vi "stim.vi"() -> ()   [LabVIEW 2010]
uses:
  <vilib>/DAQmx/write.llb/DAQmx Write (Digital Bool 1Line 1Point).vi
  Fear Conditioning/GlobalFear.vi
  <vilib>/imath/engines/lvmath2/RunTimeEngine/ErrorHandling/NIMS_Finalize Error.vi
  <vilib>/imath/engines/lvmath2/RunTimeEngine/NodeEndStatement/NIMS_NodeEndStatement_Get Vector.vi
  <instcachedir>/0/NIMS_NodeEndStatement_Get Vector_F420F1081A35401FA339BC91980782B0.lvgen/NIMS_NodeEndStatement_Get Vector_F420F1081A35401FA339BC91980782B0_002.vi
  <vilib>/imath/engines/lvmath/Functions/Error Handling/MergeErrorsWrapper.vi
  <vilib>/imath/engines/lvmath2/RunTimeEngine/NodeEndStatement/NIMS_NodeEndStatement_Output.vi
  <instcachedir>/0/NIMS_NodeEndStatement_Output_53EC0D466D134D7ABD903AC30B43404B.lvgen/NIMS_NodeEndStatement_Output_53EC0D466D134D7ABD903AC30B43404B_004.vi
  <instcachedir>/0/NIMS_NodeEndStatement_Output_53EC0D466D134D7ABD903AC30B43404B.lvgen/NIMS_NodeEndStatement_Output_53EC0D466D134D7ABD903AC30B43404B_005.vi
  <vilib>/imath/engines/lvmath2/RunTimeEngine/RangeToken/NIMS_Range.vi
  <instcachedir>/0/NIMS_Range_1C63927E4E474DADACDA97C3F2261A11.lvgen/NIMS_Range_1C63927E4E474DADACDA97C3F2261A11_000.vi
  <vilib>/imathl/engines/lvmath/Functions/Error Handling/Create Error.vi
  <vilib>/imath/engines/lvmath2/RunTimeEngine/BuiltInFunctions/repeatmx/NIMS_repeatmx(GM, I32, I32).vi
  <instcachedir>/0/NIMS_repeatmx(GM, I32, I32)_69DEE8FEFC4F4D9AB51BA55E85245ECE.lvgen/NIMS_repeatmx(GM, I32, I32)_69DEE8FEFC4F4D9AB51BA55E85245ECE_004.vi
  <vilib>/imath/engines/lvmath2/RunTimeEngine/BuiltInFunctions/randpermutation/NIMS_randpermutation.vi
  <vilib>/imath/engines/lvmath2/RunTimeEngine/VariableToken/Read/NIMS_Get Elements - SorM(_) - Check.vi
  <instcachedir>/0/NIMS_Get Elements - SorM(_) - Check_404BE36992094B78AAADB7BD5278D7E3.lvgen/NIMS_Get Elements - SorM(_) - Check_404BE36992094B78AAADB7BD5278D7E3_006.vi
  <vilib>/daqmx/miscellaneous.llb/DAQmx Fill In Error Info.vi
  <vilib>/measure/NI_MABase.lvlib
panel:
  out "Audio":bool
  in  "Audio\nSafety":bool=TRUE caption="Audio"
  out "Shock":bool
  out "Counter":dbl
  out "Elapsed Time":dbl format="%#_3g"
  out "Copleted":bool
  out "Trigger":bool
  out "Current Stim":dbl
  out "Audio\nDuration":dbl
  out "ITI":dbl
  out "Pattern \nFrequency":dbl
  out "Frequency":dbl
  out "Audio\nDelay":dbl
  out "Shock \nDuration":dbl=-1.0
  out "Shock\nDelay":dbl=-1.0
  out "raw stim":dbl
  out "Now Showing":string
  out "Dimentions":dbl
  out "expInd":dbl[](array[numeric])
  out "Stim":dbl[](array[numeric])
  out "Sum":dbl
  in  "Shock \nSafety":bool caption="Audio"
  in  "Stimuli":string[](array[combo])
  in  "Start 2":bool caption="Start"
  in  "Array 3":dbl[][](array[numeric])
  in  "Cluster 3":T1
  out "Stimulus Parameters":string[](array[string])
  in  "stop 2":bool
  # "Audio Duration"
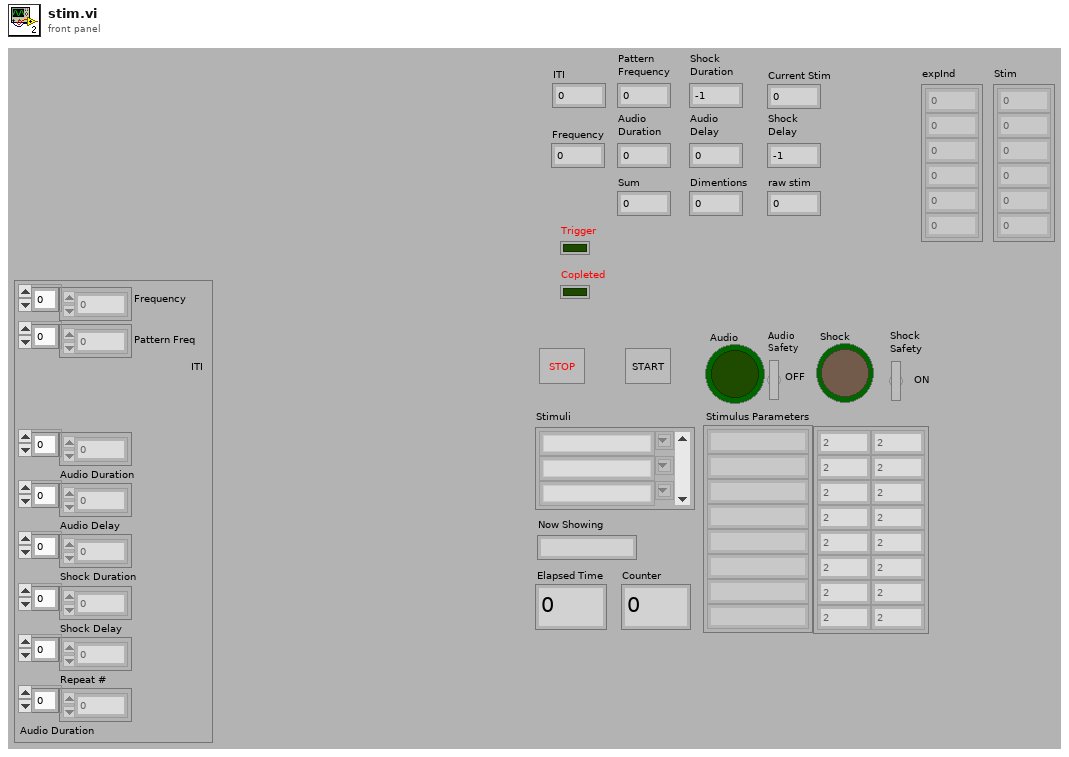
[diagram p1: front panel]
types:
  T1 = cluster{"Frequency":dbl[], "Pattern Freq":dbl[], "ITI":dbl[], "Audio Duration":dbl[], "Audio Delay":dbl[], "Shock Duration":dbl[], "Shock Delay":dbl[], "Repeat #":dbl[]}
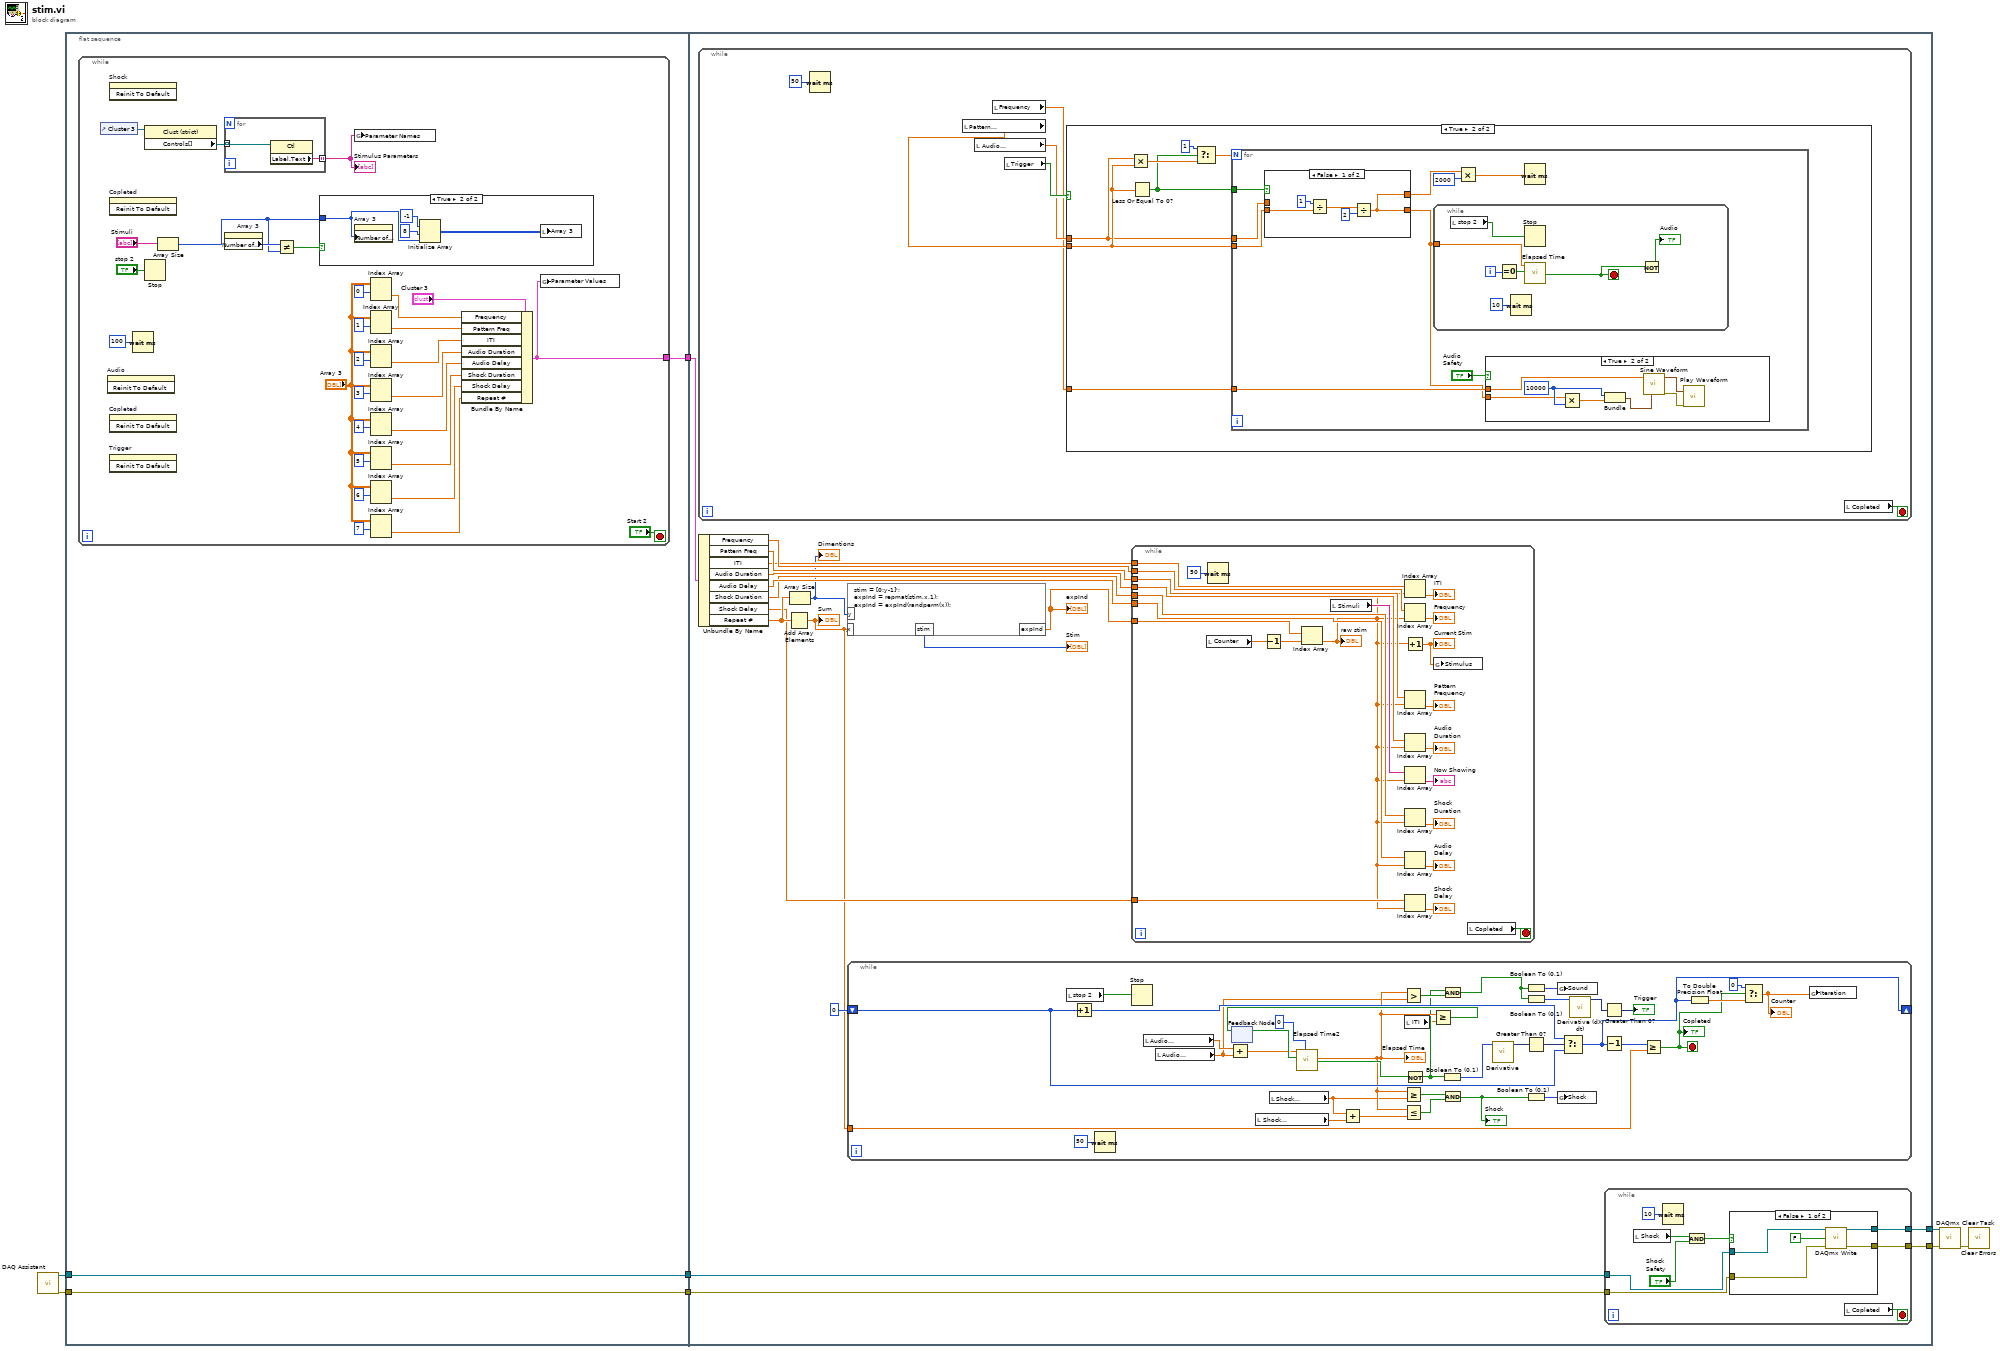
[diagram p0: block diagram]
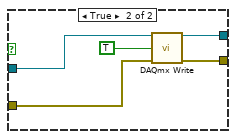
[diagram p3: hidden frame]
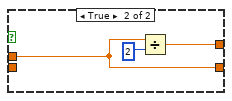
[diagram p6: hidden frame]
diagram:
  n1 = call "DAQ Assistant"() -> ("task out"=w4:refnum<k21>, "error out"=w3:errorcluster)  [unwired: 18 in]
  n2 = flat-sequence {
    tunnel: [w11] -> w8
    tunnel: w4 -> [w10]
    tunnel: [w10] -> w7
    tunnel: [w9] -> w6
    tunnel: w3 -> [w9]
    tunnel: w8 -> [w62]
    tunnel: [w50] -> w5
    tunnel: w7 -> [w49]
    tunnel: w6 -> [w48]
    tunnel: [w47] -> w2
    frame #0 {
      n3 = while {
        tunnel: [w14] -> w11
        stop <- "Start 2" stop-if-true
        n4 = control-ref of="Cluster 3"() -> (w17:refnum<vi>)
        n5 = invoke on="Audio" class="Bool (strict)" method="Reinit To Default"() -> ()  [unwired: 3 in, 3 out]
        n6 = invoke on="Shock" class="Bool (strict)" method="Reinit To Default"() -> ()  [unwired: 3 in, 3 out]
        n7 = invoke on="Copleted" class="Bool (strict)" method="Reinit To Default"() -> ()  [unwired: 3 in, 3 out]
        n8 = invoke on="Copleted" class="Bool (strict)" method="Reinit To Default"() -> ()  [unwired: 3 in, 3 out]
        n9 = invoke on="Trigger" class="Bool (strict)" method="Reinit To Default"() -> ()  [unwired: 3 in, 3 out]
        n10 = Wait (ms)(milliseconds to wait=100) -> ()  [unwired: 1 out]
        n11 = property class="Clust (strict)"(reference=w17) -> ("Controls[]"=w18:refnum<vi>[])  [unwired: 1 in, 2 out]
        n12 = Stop(stop? (T)="stop 2") -> ()
        n13 = Array Size(array="Stimuli") -> (size(s)=w39:i32)
        n14 = for {
          tunnel: [w42] -> w13 mode=indexing
          tunnel: w18 -> [w41] mode=indexing
          n15 = property class="Ctl"(reference=w41) -> ("Label.Text"=w42:string)  [unwired: 1 in, 2 out]
        }
        "Stimulus Parameters" <- w13
        n16 = property on="Array 3" class="Arr (strict)"() -> ("Number of Columns"=w40:u32)  [unwired: 2 in, 2 out]
        n17 = Not Equal?(x=w40, y=w39) -> (x != y?=w38:bool)
        n18 = case shown="True" w38 {
          tunnel: w39 -> [_ w43]
          frame False {
          }
          frame True {
            n19 = property on="Array 3" class="Arr (strict)"("Number of Columns"=w43) -> ()  [unwired: 2 in, 2 out]
            n20 = Initialize Array(-1, 8, w43) -> (w44:i32[][])
            n21 = local write "Array 3"(w44) -> ()
          }
        }
        n22 = global write "GlobalFear.vi" "Parameter Names"(w13) -> ()
        n23 = Index Array(array="Array 3", index (row)=0) -> (element=w34:dbl[])  [unwired: 1 in]
        n24 = Index Array(array="Array 3", index (row)=1) -> (element=w25:dbl[])  [unwired: 1 in]
        n25 = Index Array(array="Array 3", index (row)=2) -> (element=w24:dbl[])  [unwired: 1 in]
        n26 = Index Array(array="Array 3", index (row)=3) -> (element=w23:dbl[])  [unwired: 1 in]
        n27 = Index Array(array="Array 3", index (row)=4) -> (element=w22:dbl[])  [unwired: 1 in]
        n28 = Index Array(array="Array 3", index (row)=5) -> (element=w21:dbl[])  [unwired: 1 in]
        n29 = Index Array(array="Array 3", index (row)=6) -> (element=w20:dbl[])  [unwired: 1 in]
        n30 = Index Array(array="Array 3", index (row)=7) -> (element=w19:dbl[])  [unwired: 1 in]
        n31 = Bundle By Name(cluster="Cluster 3", "Frequency"=w34, "Pattern Freq"=w25, "ITI"=w24, "Audio Duration"=w23, "Audio Delay"=w22, "Shock Duration"=w21, "Shock Delay"=w20, "Repeat #"=w19) -> (w14:T1)
        n32 = global write "GlobalFear.vi" "Parameter Values"(w14) -> ()
      }
    }
    frame #1 {
      n33 = while {
        stop <- w210 stop-if-true
        n34 = Wait (ms)(milliseconds to wait=50) -> ()  [unwired: 1 out]
        n35 = local read "Pattern \nFrequency"() -> (w209:dbl)
        n36 = local read "Audio\nDuration"() -> (w207:dbl)
        n37 = local read "Frequency"() -> (w206:dbl)
        n38 = local read "Trigger"() -> (w208:bool)
        n39 = case shown="True" w208 {
          tunnel: w206 -> [_ w218]
          tunnel: w207 -> [_ w213]
          tunnel: w209 -> [_ w217]
          frame False {
          }
          frame True {
            n40 = Multiply(x=w213, y=w217) -> (x*y=w216:dbl)
            n41 = Less Or Equal To 0?(x=w217) -> (x <= 0?=w214:bool)
            n42 = Select(t=1, s=w214, f=w216) -> (s? t:f=w215:dbl)
            n43 = for {
              N: w215 -> [_]
              tunnel: w218 -> [w227]
              tunnel: w217 -> [w225]
              tunnel: w214 -> [w226]
              tunnel: w213 -> [w221]
              n44 = case shown="False" w226 {
                tunnel: w225 -> [w236 _]
                tunnel: [w235 w242] -> w220
                tunnel: [w235 w240] -> w222
                tunnel: w221 -> [_ w242]
                frame False {
                  n45 = Divide(x=1, y=w236) -> (x/y=w237:dbl)
                  n46 = Divide(x=w237, y=2) -> (x/y=w235:dbl)
                }
                frame True {
                  n47 = Divide(x=w242, y=2) -> (x/y=w240:dbl)
                }
              }
              n48 = while {
                tunnel: w220 -> [w249]
                i -> [w248]
                stop <- w245 stop-if-true
                n49 = local read "stop 2"() -> (w243:bool)
                n50 = Equal To 0?(x=w248) -> (x = 0?=w247:bool)
                n51 = Wait (ms)(milliseconds to wait=10) -> ()  [unwired: 1 out]
                n52 = Stop(stop? (T)=w243) -> ()
                n53 = call "Elapsed Time"("Time Target (s)"=w249, "Reset"=w247) -> ("Time has Elapsed"=w245:bool)  [unwired: 10 in, 7 out]
                n54 = Not(x=w245) -> (.not. x?=→"Audio":bool)
              }
              n55 = Multiply(x=w222, y=2000) -> (x*y=w224:dbl)
              n56 = case shown="True" "Audio\nSafety" {
                tunnel: w227 -> [_ w234]
                tunnel: w220 -> [_ w228]
                frame False {
                }
                frame True {
                  w233 = 10000
                  n57 = Multiply(x=w228, y=w233) -> (x*y=w232:dbl)
                  n58 = Bundle(w233, w232) -> (w231:cluster{i32, dbl})  [unwired: 1 in]
                  n59 = call <vilib>:"Sine Waveform.vi"("sampling info"=w231, "frequency"=w234) -> ("error out"=w229:errorcluster, "signal out"=w230:waveform(dbl))  [unwired: 8 in]
                  n60 = call "Play Waveform"("Data"=w230, "error in"=w229) -> ()  [unwired: 17 in, 1 out]
                }
              }
              n61 = Wait (ms)(milliseconds to wait=w224) -> ()  [unwired: 1 out]
            }
          }
        }
        n62 = local read "Copleted"() -> (w210:bool)
      }
      n63 = Unbundle By Name(w62) -> ("Frequency"=w61:dbl[], "Pattern Freq"=w60:dbl[], "ITI"=w59:dbl[], "Audio Duration"=w58:dbl[], "Audio Delay"=w57:dbl[], "Shock Duration"=w56:dbl[], "Shock Delay"=w55:dbl[], "Repeat #"=w63:dbl[])
      n64 = Add Array Elements(numeric array=w63) -> (sum=w51:dbl)
      "Sum" <- w51
      n65 = Array Size(array=w63) -> (size(s)=w54:i32)
      "Dimentions" <- w54
      n66 = mathscript code="stim = [0:y-1]';\nexpInd = repmat(stim,x,1);\nexpInd = expInd(randperm(x));"("x"=w51, "y"=w54) -> ("expInd"=w53:dbl[], "stim"=→"Stim":i32[])  [unwired: 1 in, 1 out]
      "expInd" <- w53
      n67 = while {
        shift-right: [w179] -> _
        shift-left: 0 -> [w193]
        tunnel: w51 -> [w177]
        stop <- w181 stop-if-true
        n68 = local read "stop 2"() -> (w175:bool)
        n69 = Increment(x=w193) -> (x+1=w194:i32)
        n70 = Wait (ms)(milliseconds to wait=50) -> ()  [unwired: 1 out]
        n71 = Stop(stop? (T)=w175) -> ()
        n72 = local read "Audio\nDuration"() -> (w173:dbl)
        n73 = local read "Audio\nDelay"() -> (w171:dbl)
        n74 = Add(x=w173, y=w171) -> (x+y=w190:dbl)
        n75 = feedback #1() -> (w199:bool)  [unwired: 1 in]
        n76 = local read "Shock \nDuration"() -> (w169:dbl)
        n77 = local read "Shock\nDelay"() -> (w170:dbl)
        n78 = call "Elapsed Time2"("Time Target (s)"=w190, "Reset"=w199, "Set Start Time (s)"=0) -> ("Elapsed Time (s)"=w187:dbl, "Time has Elapsed"=w200:bool)  [unwired: 9 in, 6 out]
        "Elapsed Time" <- w187
        n79 = Add(x=w170, y=w169) -> (x+y=w203:dbl)
        n80 = Greater?(x=w187, y=w171) -> (0:w188:bool)
        n81 = Greater Or Equal?(x=w187, y=w170) -> (x >= y?=w202:bool)
        n82 = Less Or Equal?(x=w187, y=w203) -> (x <= y?=w204:bool)
        n83 = local read "ITI"() -> (w172:dbl)
        n84 = Not(x=w200) -> (.not. x?=w184:bool)
        n85 = Greater Or Equal?(x=w187, y=w172) -> (x >= y?=w195:bool)
        n86 = feedback-in #1(w195) -> ()
        n87 = Boolean To (0,1)(Boolean=w184) -> (0, 1=w186:i16)
        n88 = And(x=w184, y=w188) -> (x .and. y?=w189:bool)
        n89 = And(x=w202, y=w204) -> (x .and. y?=w174:bool)
        "Shock" <- w174
        n90 = call "Derivative"("Signals"=w186) -> ("Result"=w185:dynamicdata)  [unwired: 5 in, 1 out]
        n91 = Boolean To (0,1)(Boolean=w189) -> (0, 1=w191:i16)
        n92 = Boolean To (0,1)(Boolean=w189) -> (0, 1=w198:i16)
        n93 = Greater Than 0?(x=w185) -> (x > 0?=w183:dynamicdata)
        n94 = Boolean To (0,1)(Boolean=w174) -> (0, 1=w192:i16)
        n95 = global write "GlobalFear.vi" "Sound"(w191) -> ()
        n96 = global write "GlobalFear.vi" "Shock"(w192) -> ()
        n97 = Select(t=w194, s=w183, f=w193) -> (s? t:f=w179:i32)
        n98 = call "Derivative (dX/dt)"("Signals"=w198) -> ("Result"=w197:dynamicdata)  [unwired: 5 in, 1 out]
        n99 = Greater Than 0?(x=w197) -> (x > 0?=→"Trigger":dynamicdata)
        n100 = Decrement(x=w179) -> (x-1=w178:i32)
        n101 = Greater Or Equal?(x=w178, y=w177) -> (x >= y?=w181:bool)
        "Copleted" <- w181
        n102 = To Double Precision Float(number=w179) -> (double precision float=w182:dbl)
        n103 = Select(t=0, s=w181, f=w182) -> (s? t:f=w176:dbl)
        "Counter" <- w176
        n104 = global write "GlobalFear.vi" "Iteration"(w176) -> ()
      }
      n105 = while {
        tunnel: w53 -> [w105]
        tunnel: w61 -> [w104]
        tunnel: w60 -> [w103]
        tunnel: w59 -> [w102]
        tunnel: w58 -> [w101]
        tunnel: w57 -> [w95]
        tunnel: w56 -> [w92]
        tunnel: w55 -> [w91]
        stop <- w106 stop-if-true
        n106 = local read "Counter"() -> (w89:dbl)
        n107 = Wait (ms)(milliseconds to wait=50) -> ()  [unwired: 1 out]
        n108 = Decrement(x=w89) -> (x-1=w90:dbl)
        n109 = Index Array(array=w105, index=w90) -> (element=w86:dbl)
        "raw stim" <- w86
        n110 = local read "Stimuli"() -> (w87:string[])
        n111 = Index Array(array=w102, index=w86) -> (element=→"ITI":dbl)
        n112 = Index Array(array=w104, index=w86) -> (element=→"Frequency":dbl)
        n113 = Increment(x=w86) -> (x+1=w84:dbl)
        "Current Stim" <- w84
        n114 = Index Array(array=w103, index=w86) -> (element=→"Pattern \nFrequency":dbl)
        n115 = Index Array(array=w101, index=w86) -> (element=→"Audio\nDuration":dbl)
        n116 = Index Array(array=w87, index=w86) -> (element=→"Now Showing":string)
        n117 = Index Array(array=w92, index=w86) -> (element=→"Shock \nDuration":dbl)
        n118 = Index Array(array=w95, index=w86) -> (element=→"Audio\nDelay":dbl)
        n119 = Index Array(array=w91, index=w86) -> (element=→"Shock\nDelay":dbl)
        n120 = global write "GlobalFear.vi" "Stimulus"(w84) -> ()
        n121 = local read "Copleted"() -> (w106:bool)
      }
      n122 = while {
        tunnel: [w73] -> w50
        tunnel: w49 -> [w70]
        tunnel: w48 -> [w69]
        tunnel: [w68] -> w47
        stop <- w71 stop-if-true
        n123 = local read "Shock"() -> (w66:bool)
        n124 = Wait (ms)(milliseconds to wait=10) -> ()  [unwired: 1 out]
        n125 = And(x=w66, y="Shock \nSafety") -> (x .and. y?=w67:bool)
        n126 = case shown="False" w67 {
          tunnel: [w77 w82] -> w73
          tunnel: w70 -> [w76 w81]
          tunnel: w69 -> [w74 w80]
          tunnel: [w75 w79] -> w68
          frame False {
            n127 = call-poly <vilib>:"DAQmx Write.vi"("task/channels in"=w76, "data"=FALSE, "error in"=w74) -> ("task out"=w77:refnum<k21>, "error out"=w75:errorcluster)  [unwired: 10 in, 1 out]
          }
          frame True {
            n128 = call-poly <vilib>:"DAQmx Write.vi"("task/channels in"=w81, "data"=TRUE, "error in"=w80) -> ("task out"=w82:refnum<k21>, "error out"=w79:errorcluster)  [unwired: 10 in, 1 out]
          }
        }
        n129 = local read "Copleted"() -> (w71:bool)
      }
    }
  }
  n130 = call <vilib>:"DAQmx Clear Task.vi"("task in"=w5, "error in"=w2) -> ("error out"=w1:errorcluster)  [unwired: 13 in]
  n131 = call <vilib>:"Clear Errors.vi"("error in (no error)"=w1) -> ()  [unwired: 6 in, 1 out]
